vi "Grove Digital Out.vi"() -> ()   [LabVIEW 2020, in "CTI-Scratchpad.lvlib"]
uses:
  CTI-Scratchpad.lvlib
  CTI/Identity.ctl
  CTI/GPIO Direction.ctl
  CTI/GPIO Number.ctl
  CTI/Session/Session.lvclass
  CTI/CTI.lvlib
  CTI/VisaComms/VisaComms.lvclass
panel:
  out "Readback1":bool
  in  "GroveConnector":enum16{"D16", "D18", "D20"}(ring)
  out "Identity":T1
  in  "Control":bool
  in  "Port":refnum<visa-resource-name>="COM6"
  in  "stop":bool
  # "https://wiki.seeedstudio.com/Grove-Relay/"
  # "https://wiki.seeedstudio.com/Grove-EL_Driver/"
  # "https://wiki.seeedstudio.com/Grove-Electromagnet/"
  # "https://wiki.seeedstudio.com/Grove-Mini_Fan/"
  # "https://wiki.seeedstudio.com/Grove-Infrared_Emitter/"
  # "https://wiki.seeedstudio.com/Grove-Optocoupler_Relay-M281/"
  # "https://wiki.seeedstudio.com/Grove-Solid_State_Relay/"
  # "https://wiki.seeedstudio.com/Grove-Solid_State_Relay_V2/"
  # "https://wiki.seeedstudio.com/Grove-SPDT_Relay_30A/"
  # "https://wiki.seeedstudio.com/Grove-Vibration_Motor/"
  # "https://wiki.seeedstudio.com/Grove-2-Channel_SPDT_Relay/"
  # "https://wiki.seeedstudio.com/Grove-Relay/"
  # "https://wiki.seeedstudio.com/Grove-LED_Socket_Kit/"
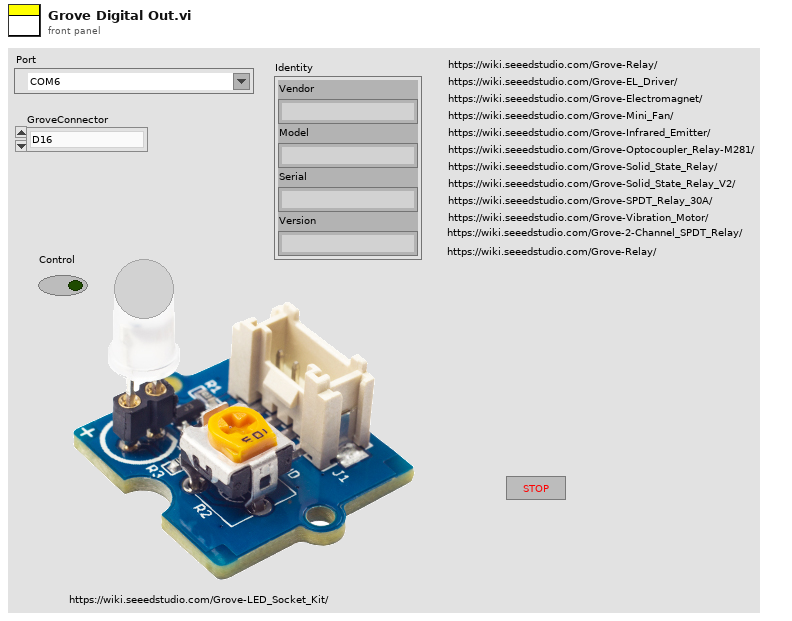
[diagram p1: front panel]
types:
  T1 = typedef "CTI.lvlib/Identity.ctl" = cluster{"Vendor":string, "Model":string, "Serial":string, "Version":string}
  T2 = typedef "CTI.lvlib/GPIO Direction.ctl" = enum16{"In", "Out"}
  T3 = typedef "CTI.lvlib/GPIO Number.ctl" = i8
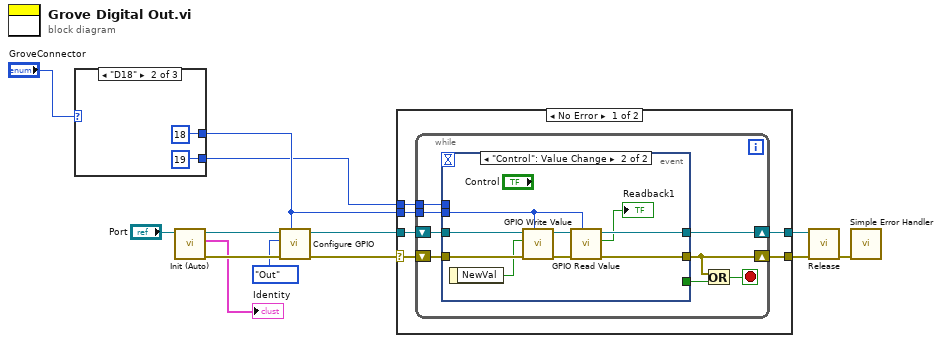
[diagram p0: block diagram]
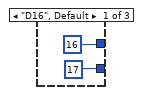
[diagram p2: hidden frame]
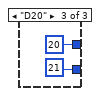
[diagram p3: hidden frame]
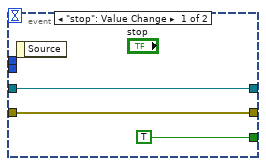
[diagram p4: hidden frame]
diagram:
  n1 = case shown="\"D18\"" "GroveConnector" {
    tunnel: [T3 16 ("GPIO #") T3 18 ("GPIO #") T3 20 ("GPIO #")] -> w4
    tunnel: [T3 17 ("GPIO #") T3 19 ("GPIO #") T3 21 ("GPIO #")] -> w3
    frame "D16", Default {
    }
    frame "D18" {
    }
    frame "D20" {
    }
  }
  n2 = call "Init (Auto).vi"("VISA resource name"="Port") -> ("error out"=w11:errorcluster, "Identity"=→"Identity":T1, "Session"=w12:refnum<class "Session.lvclass">)  [unwired: 8 in]
  n3 = call "Configure GPIO.vi"("GPIO #"=w4, "error in (no error)"=w11, "GPIO Direction"=GPIO_Direction."Out", "Session in"=w12) -> ("error out"=w1:errorcluster, "Session out"=w2:refnum<class "Session.lvclass">)  [unwired: 6 in]
  n4 = case shown="No Error" w1 {
    selector: w1 -> [w24 w46]
    tunnel: w2 -> [w25 w47]
    tunnel: [w23 w47] -> w8
    tunnel: [w22 w46] -> w10
    tunnel: w4 -> [w21 _]
    tunnel: w3 -> [w20 _]
    frame No Error {
      n5 = while {
        shift-right: [w31] -> w23
        shift-left: w25 -> [w33]
        shift-right: [w30] -> w22
        shift-left: w24 -> [w32]
        tunnel: w21 -> [w27]
        tunnel: w20 -> [w26]
        stop <- w29 stop-if-true
        n6 = event shown="[1] \"Control\": Value Change" {
          selector: _ -> [_ _]
          dyn-events: _ -> [_ _]
          timeout: _ -> [_ _]
          tunnel: w33 -> [w36 w45]
          tunnel: w32 -> [w35 w44]
          tunnel: [w36 w43] -> w31
          tunnel: [w35 w42] -> w30
          tunnel: [TRUE _] -> w28
          tunnel: w27 -> [_ w39]
          tunnel: w26 -> [_ _]
          event "stop": Value Change {
            n7 = event-data() -> ()  [unwired: 1 in, 1 out]
          }
          event "Control": Value Change {
            n8 = event-data() -> ("NewVal"=w38:bool)  [unwired: 1 in]
            n9 = call "GPIO Write Value.vi"("GPIO #"=w39, "error in (no error)"=w44, "Value"=w38, "Session in"=w45) -> ("error out"=w40:errorcluster, "Session out"=w41:refnum<class "Session.lvclass">)  [unwired: 6 in]
            n10 = call "GPIO Read Value.vi"("GPIO #"=w39, "error in (no error)"=w40, "Session in"=w41) -> ("error out"=w42:errorcluster, "Value"=→"Readback1":bool, "Session out"=w43:refnum<class "Session.lvclass">)  [unwired: 6 in]
          }
        }
        n11 = Or(x=w30, y=w28) -> (x .or. y?=w29:bool)
      }
    }
    frame Error {
    }
  }
  n12 = call-dynamic "Release.vi"("error in (no error)"=w10, "Session in"=w8) -> ("error out"=w9:errorcluster)  [unwired: 9 in]
  n13 = call <vilib>:"Simple Error Handler.vi"("error in (no error)"=w9) -> ()  [unwired: 4 in, 5 out]
